vi "Sr830 ErrorHandler.vi"(8 "error in (no error)":errorcluster caption="entrée d'erreur (pas d'erreur)", 10 "Pass Error":bool caption="PassError(F)", 11 "VisaRes":refnum<visa-resource-name>) -> (0 "error out":errorcluster caption="sortie d'erreur", 3 "message":string=" INSTRUCTIONS:\r\rNormal Use:  When using subVIs that incorporate the error in/error out (or error I/O) structure, place this handler where you want to inform the user of an error, typically at the end of the I/O data path, as the last action of the program.  If the error in error? is ERROR, the handler creates a message describing the error and its source.  If the type of dialog = 1 (default), the message is displayed to the user, who can only acknowedge it.  If the type = 2, the user can acknowledge the message or abort execution; aborting a program with active I/O is not recommended.  If the type = 0, no message is displayed; this is used to process the error programmatically, and the error out cluster elements are wired to individual terminals for that reason.  \r\rOther Use:\n\r\nlocal testing.  To test the error code of a subVI or function that does not have the error I/O structure, you can wire its error code and a source string to the local error code and error source inputs.  If error in error? indicates no error and error code is not equal to 0, the local code and source are substituted for the error in values, and error? is set TRUE (ERROR).")   [LabVIEW 2019]
uses:
  <vilib>/Utility/error.llb/DialogType.ctl
panel:
  in  "stop":bool
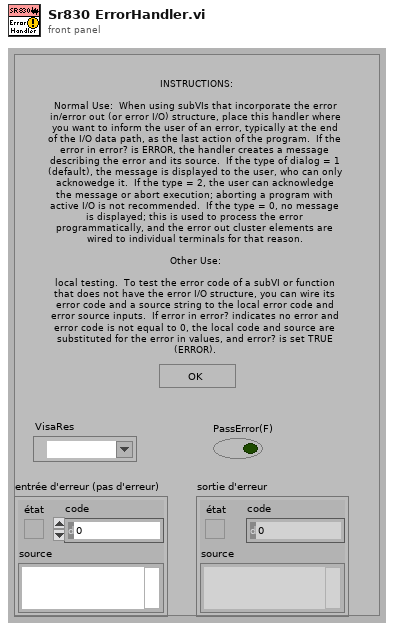
[diagram p1: front panel]
types:
  T1 = enum32{"Invalid", "Standard", "Closed", "Hidden", "Minimized", "Maximized"}
  T2 = typedef "DialogType.ctl" = u16
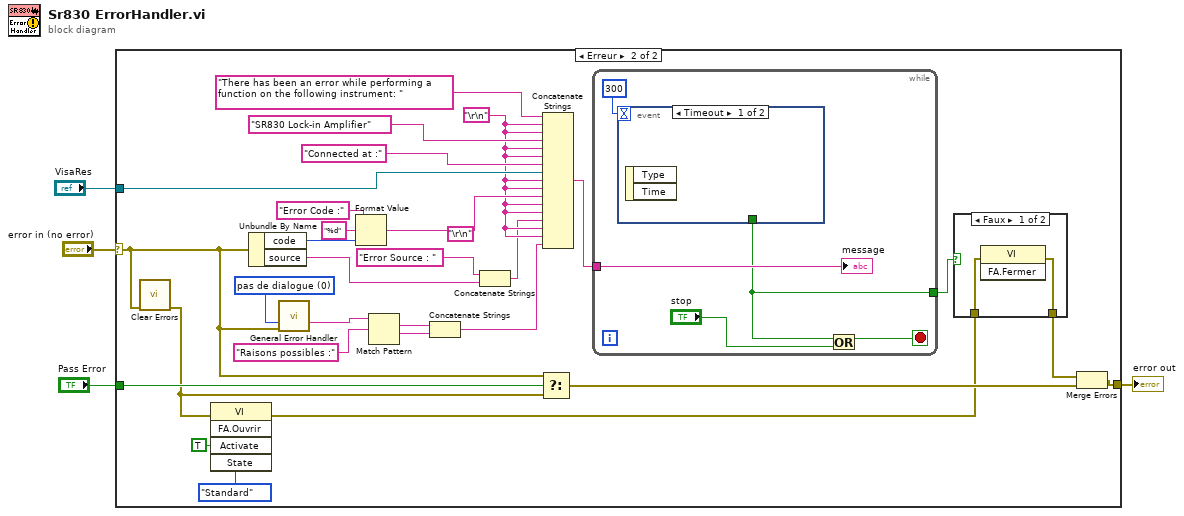
[diagram p0: block diagram]
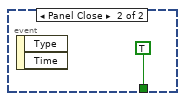
[diagram p4: hidden frame]
diagram:
  n1 = case shown="Erreur" "error in (no error)" {
    selector: "error in (no error)" -> [w5 w11]
    tunnel: "VisaRes" -> [_ w31]
    tunnel: [w5 w8] -> w3
    tunnel: "Pass Error" -> [_ w26]
    frame No Error {
    }
    frame Error {
      (unwired) "\r\n"
      w21 = T2 0 items=["pas de dialogue", "Message OK", "Message continuer ou arrêter", "Message OK + mises en garde", "Arrêter/Continuer + mises en garde"] ("type of dialog (OK msg:1)")
      w20 = "\r\n"
      n2 = call <vilib>:"Clear Errors.vi"("error in (no error)"=w11) -> ("error out"=w10:errorcluster)  [unwired: 5 in, 1 out]
      n3 = invoke class="VI" method="FA.Ouvrir"(error in=w10, "Activate"=TRUE ("Activer ?"), "State"=T1."Standard" ("État")) -> (error out=w6:errorcluster)  [unwired: 2 in, 4 out]
      n4 = Unbundle By Name(w11) -> ("code"=w34:i32, "source"=w28:string)
      n5 = call <vilib>:"General Error Handler.vi"("type of dialog (OK msg:1)"=w21, "error in (no error)"=w11) -> ("message"=w18:string)  [unwired: 9 in, 4 out]
      n6 = Format Value(string ("")="Error Code :" ("chaîne (\"\")"), format string="%d" ("chaîne de format"), value (0)=w34) -> (output string=w30:string)
      n7 = Match Pattern(string=w18, regular expression="Raisons possibles :" ("message")) -> (match substring=w16:string, after substring=w15:string)  [unwired: 1 in, 2 out]
      n8 = Concatenate Strings(w16, w15) -> (w14:string)
      n9 = Concatenate Strings("Error Source : " ("chaîne (\"\")"), w28) -> (w19:string)
      n10 = Select(t=w11, s=w26, f=w10) -> (s? t:f=w9:errorcluster)
      n11 = Concatenate Strings("There has been an error while performing a function on the following instrument: " ("message"), w20, w20, "SR830 Lock-in Amplifier" ("message"), w20, w20, "Connected at :" ("message"), w31, w20, w20, w30, w20, w20, w19, w20, w20, w14) -> (w27:string)
      n12 = while {
        tunnel: w27 -> [w42]
        tunnel: [w38] -> w22
        stop <- w40 stop-if-true
        n13 = event shown="[0] Timeout" {
          selector: _ -> [_ _]
          dyn-events: _ -> [_ _]
          timeout: u32 300 ("milliseconds to wait") -> [_ _]
          tunnel: [_ TRUE] -> w38
          event Timeout {
            n14 = event-data() -> ()  [unwired: 1 in, 2 out]
          }
          event Panel Close {
            n15 = event-data() -> ()  [unwired: 1 in, 2 out]
          }
        }
        n16 = Or(x=w38, y="stop") -> (x .or. y?=w40:bool)
        "message" <- w42
      }
      n17 = case shown="Faux" w22 {
        tunnel: w6 -> [w36 w37]
        tunnel: [w35 w37] -> w7
        frame False {
          n18 = invoke class="VI" method="FA.Fermer"(error in=w36) -> (error out=w35:errorcluster)  [unwired: 2 in, 2 out]
        }
        frame True {
        }
      }
      n19 = Merge Errors(w7, w9) -> (w8:errorcluster)
    }
  }
  "error out" <- w3
